vi "Labviewmain.vi"() -> ()   [LabVIEW 2024]
uses:
  029cd170-5375-4eb0-abf1-af2798c973fd.vi
  <vilib>/measure/NI_MABase.lvlib
panel:
  out "Array":dbl[][](array[numeric])
  out "data 2":dynamicdata(graph) caption="data"
  in  "sampling info":cluster{"Fs":dbl, "#s":dbl}={"Fs"=1000.0, "#s"=1000.0} {"Fs" format="%.2p"}
  in  "amplitude":dbl=1.0 format="%0.2p"
  in  "frequency":dbl=10.0 format="%0.2p"
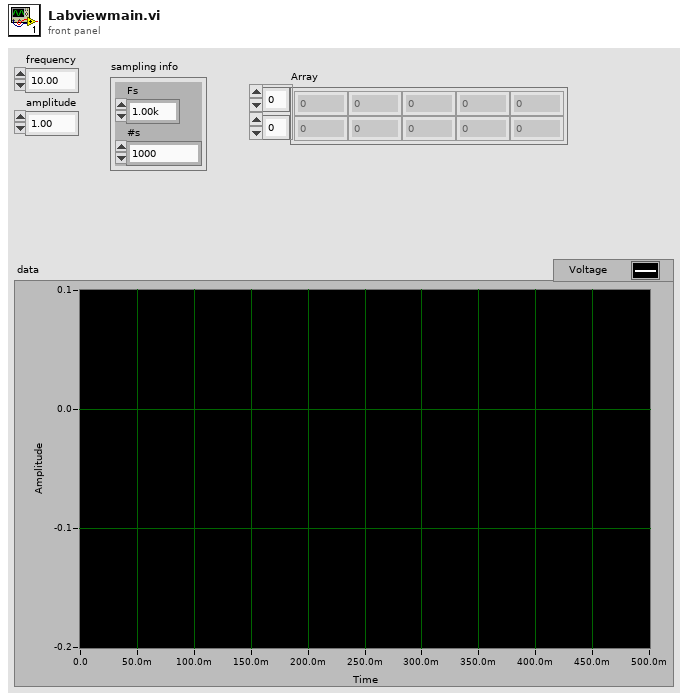
[diagram p1: front panel]
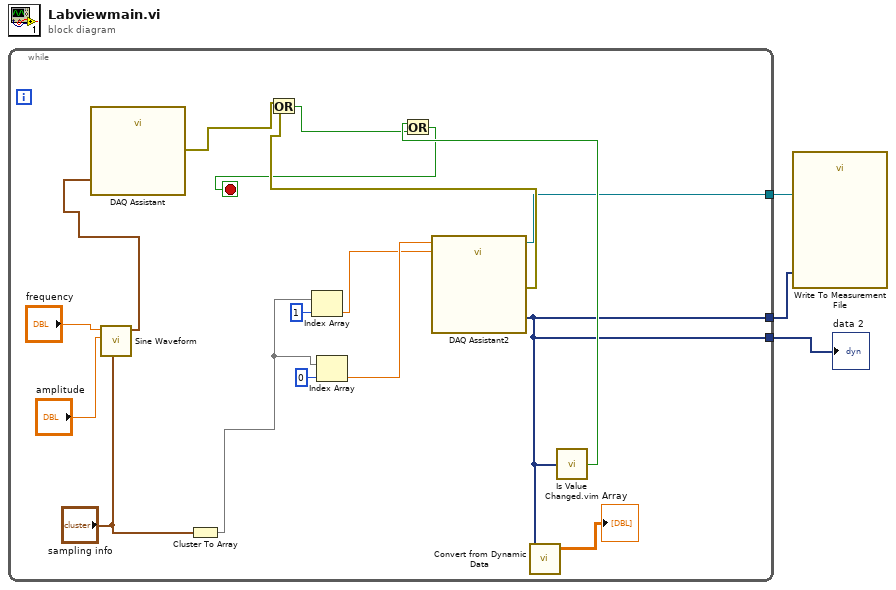
[diagram p0: block diagram]
diagram:
  n1 = while {
    tunnel: [w5] -> w3
    tunnel: [w5] -> w2
    tunnel: [w4] -> w1
    stop <- w16 stop-if-true
    n2 = call <vilib>:"Sine Waveform.vi"("sampling info"="sampling info", "amplitude"="amplitude", "frequency"="frequency") -> ("signal out"=w14:waveform(dbl))  [unwired: 7 in, 1 out]
    n3 = call "DAQ Assistant"("data"=w14) -> ("error out"=w13:errorcluster)  [unwired: 16 in, 2 out]
    n4 = Cluster To Array(cluster="sampling info") -> (array=w10:dbl[])
    n5 = Index Array(array=w10, index=1) -> (element=w6:dbl)
    n6 = Index Array(array=w10, index=0) -> (element=w7:dbl)
    n7 = call "DAQ Assistant2"("rate"=w7, "number of samples"=w6) -> ("task out"=w4:refnum<k21>, "data"=w5:dynamicdata, "error out"=w19:errorcluster)  [unwired: 14 in, 1 out]
    n8 = Or(x=w13, y=w19) -> (x .or. y?=w17:bool)
    n9 = call "Convert from Dynamic Data"("Dynamic Data Type"=w5) -> ("Array"=→"Array":dbl[][])  [unwired: 3 in]
    n10 = call "Is Value Changed.vim"("value"=w5) -> ("changed or first call?"=w18:bool)
    n11 = Or(x=w18, y=w17) -> (x .or. y?=w16:bool)
  }
  "data 2" <- w3
  n12 = call "Write To Measurement File"("Signals"=w2, "DAQmx Task"=w1) -> ()  [unwired: 15 in, 3 out]
